vi "Test Nested Read Linker Info.vi"(8 "error in (no error)":errorcluster) -> (0 "error out":errorcluster)   [LabVIEW 2013]
uses:
  classes/Test Runner.Folder/Test Runner.Folder.lvclass
  classes/Assert/Assert.lvclass
  classes/Test/Test.lvclass
panel:
  out "Test VIs":path[](array[path])
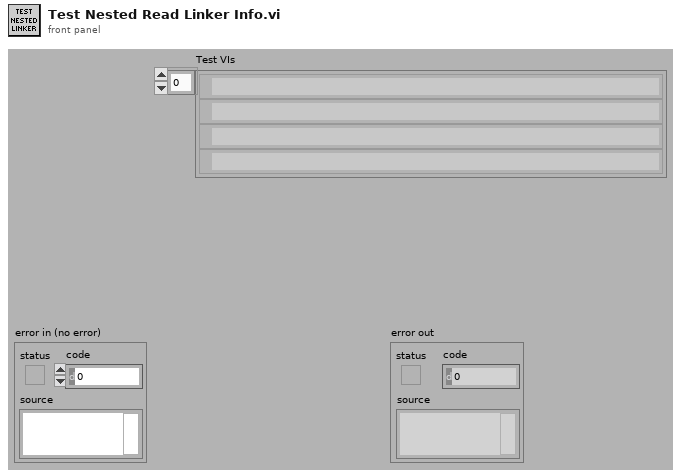
[diagram p1: front panel]
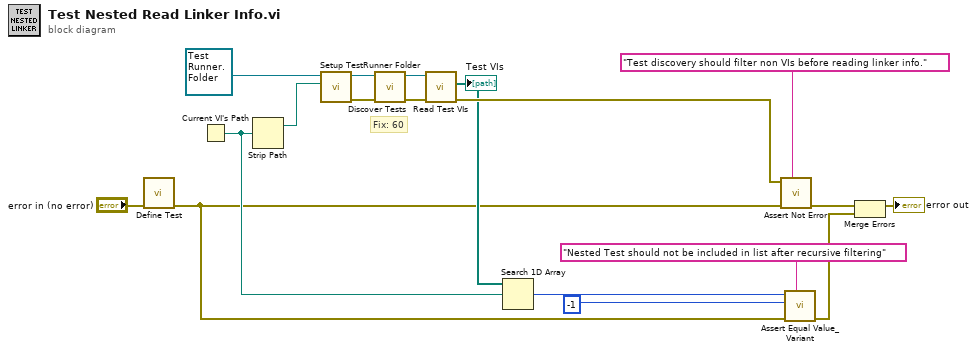
[diagram p0: block diagram]
diagram:
  # "Fix: 60"
  n1 = call "Define Test.vi"("error in (no error)"="error in (no error)") -> ("error out"=w9:errorcluster)  [unwired: 10 in]
  n2 = Current VI's Path() -> (path=w10:path)
  n3 = Strip Path(path=w10) -> (stripped path=w4:path)  [unwired: 1 out]
  n4 = call "Setup TestRunner Folder.vi"("Directory to search"=w4, "Test Runner.Folder"=refnum<class "Test Runner.Folder.lvclass"> refnum ("Caraya.lvlib:Test Runner.Folder.lvclass")) -> ("error out"=w2:errorcluster, "Test Runner.Folder out"=w3:refnum<class "Test Runner.Folder.lvclass">)  [unwired: 8 in]
  n5 = call-dynamic "Discover Tests.vi"("error in (no error)"=w2, "Test Runner in"=w3) -> ("error out"=w14:errorcluster, "Test Runner out"=w12:refnum<class "Test Runner.Folder.lvclass">)  [unwired: 8 in]
  n6 = call-dynamic "Read Test VIs.vi"("error in (no error)"=w14, "Test Runner in"=w12) -> ("error out"=w13:errorcluster, "Test VIs"=w11:path[])  [unwired: 7 in, 1 out]
  "Test VIs" <- w11
  n7 = Search 1D Array(1D array=w11, element=w10) -> (index of element=w6:i32)  [unwired: 1 in]
  n8 = call "Assert Not Error.vi"("Label"="Test discovery should filter non VIs before reading linker info.", "error in (no error)"=w9, "Not Error?"=w13) -> ("error out"=w16:errorcluster)  [unwired: 8 in]
  n9 = call "Assert Equal Value_Variant.vi"("Label"="Nested Test should not be included in list after recursive filtering", "error in (no error)"=w9, "Y"=-1 ("index of element"), "X"=w6) -> ("error out"=w8:errorcluster)  [unwired: 7 in]
  n10 = Merge Errors(w16, w8) -> (→"error out":errorcluster)
